vi "XML429_Channel_GetChannels.vi"(0 "BoardConfig in":refnum<k20>, 11 "Error in":errorcluster) -> (4 "BoardConfig out":refnum<k20>, 6 "Channels":refnum<k20>[](array[refnum]), 15 "Error out":errorcluster)   [LabVIEW 2016]
doc: "XML429_Channel_GetChannels"
uses:
  <vilib>/xml/NI_XML.lvlib
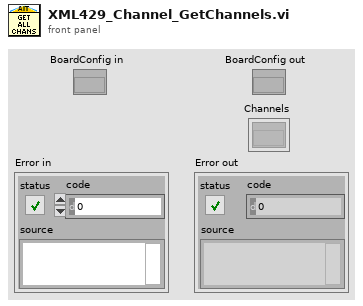
[diagram p1: front panel]
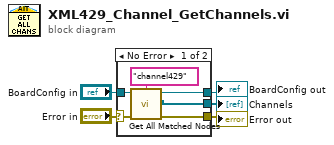
[diagram p0: block diagram]
diagram:
  n1 = case shown="No Error" "Error in" {
    selector: "Error in" -> [w11 w13]
    tunnel: [w8 w13] -> w4
    tunnel: "BoardConfig in" -> [w10 w12]
    tunnel: [w6 w12] -> w2
    tunnel: [w7 _] -> w1
    frame No Error {
      n2 = call <vilib>:"Get All Matched Nodes.vi"("error in (no error)"=w11, "XPath expression"="channel429", "node in"=w10) -> ("error out"=w8:errorcluster, "node result array"=w7:refnum<k20>[], "node out"=w6:refnum<k20>)  [unwired: 6 in]
    }
    frame Error {
    }
  }
  "Error out" <- w4
  "BoardConfig out" <- w2
  "Channels" <- w1
